vi "Import data part 1.vi"() -> (1 "New Qs":T1[](array[typedef]), 3 "canceled?":bool)   [LabVIEW 2013]
uses:
  TD - Data type.ctl
  qwtblvlib/TD Quantity.ctl
  qwtblvlib/QWTBLVLib.lvlib
panel:
  in  "note":string="This vi can import only from csv/dat files."
  out "data type":T2
  in  "next":bool
  in  "Cancel":bool
  in  "Data filename":path
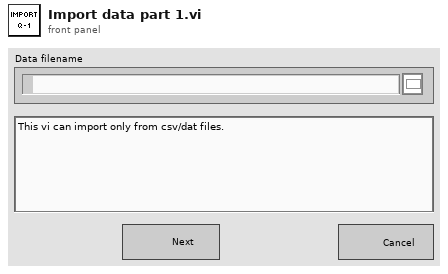
[diagram p1: front panel]
types:
  T1 = typedef "QWTBLVLib.lvlib/TD Quantity.ctl" = cluster{"Name":string, "Value":dbl[][], "Uncertainty":dbl[][], "Degrees of Freedom":dbl[][], "Correlation":dbl[][], "Randomized uncertainty":dbl[][]}
  T2 = typedef "TD - Data type.ctl" = enum32{"unknown", "csv", "xls/xlsx"}
  T3 = enum8{"Enabled", "Disabled", "Disabled and Grayed Out"}
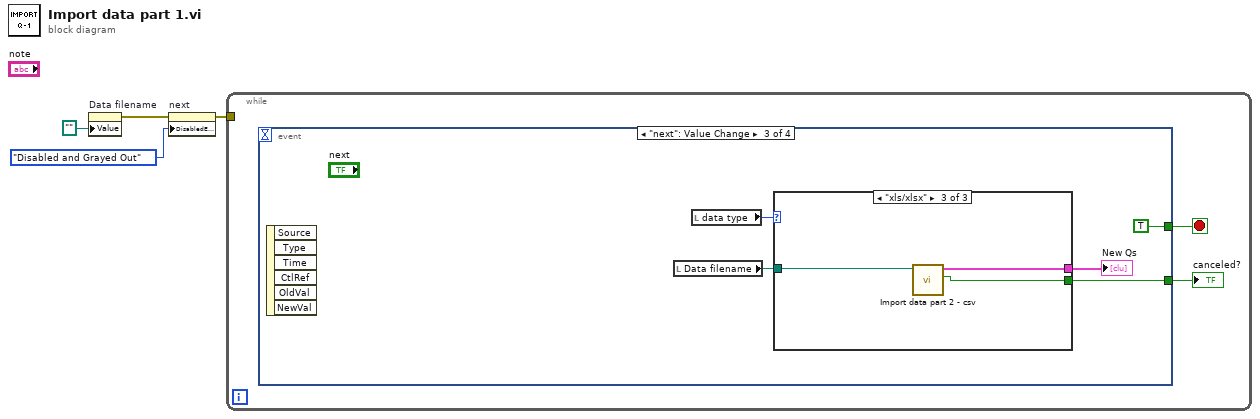
[diagram p0: block diagram]
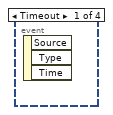
[diagram p2: hidden frame]
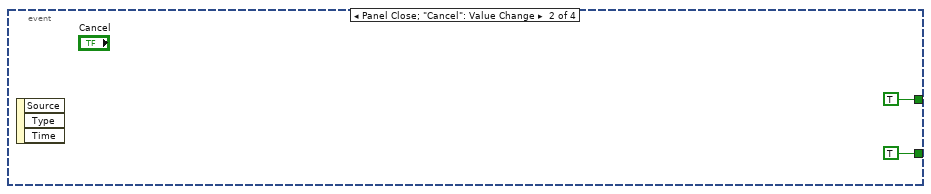
[diagram p3: hidden frame]
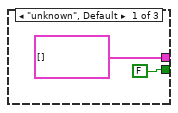
[diagram p4: hidden frame]
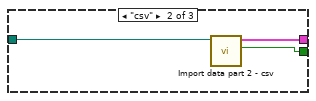
[diagram p5: hidden frame]
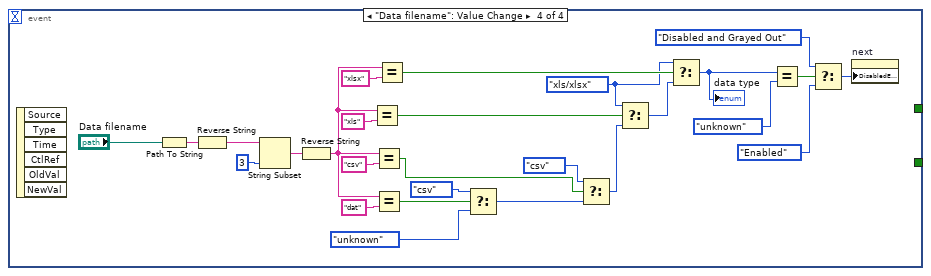
[diagram p6: hidden frame]
diagram:
  n1 = property on="Data filename" class="Path"("Value"=path "") -> (error out=w1:errorcluster)  [unwired: 2 in, 1 out]
  n2 = property on="next" class="Bool"(error in=w1, "DisabledEnum"=T3."Disabled and Grayed Out" ("Disabled")) -> (error out=w3:errorcluster)  [unwired: 1 in, 1 out]
  n3 = while {
    tunnel: w3 -> [_]
    stop <- w6 stop-if-true
    n4 = event shown="[2] \"next\": Value Change" {
      selector: _ -> [_ _ _ _]
      dyn-events: _ -> [_ _ _ _]
      timeout: _ -> [_ _ _ _]
      tunnel: [_ TRUE TRUE _] -> w6
      tunnel: [_ TRUE ("canceled") w10 _] -> w5
      event Timeout {
        n5 = event-data() -> ()  [unwired: 1 in, 3 out]
      }
      event Panel Close; "Cancel": Value Change {
        n6 = event-data() -> ()  [unwired: 1 in, 3 out]
      }
      event "next": Value Change {
        n7 = event-data() -> ()  [unwired: 1 in, 6 out]
        n8 = local read "Data filename"() -> (w13:path)
        n9 = local read "data type"() -> (w11:T2)
        n10 = case shown="\"xls/xlsx\"" w11 {
          tunnel: w13 -> [_ w18 w21]
          tunnel: [T1[] [] ("New Qs") w17 w20] -> w9
          tunnel: [FALSE ("canceled?") w16 w19] -> w10
          frame "unknown", Default {
          }
          frame "csv" {
            n11 = call "Import data part 2 - csv.vi"("Data filename"=w18) -> ("canceled?"=w16:bool, "New Qs"=w17:T1[])  [unwired: 7 in]
          }
          frame "xls/xlsx" {
            n12 = call "Import data part 2 - csv.vi"("Data filename"=w21) -> ("canceled?"=w19:bool, "New Qs"=w20:T1[])  [unwired: 7 in]
          }
        }
        "New Qs" <- w9
      }
      event "Data filename": Value Change {
        w31 = TD_-_Data_type."xls/xlsx" ("data type")
        n13 = event-data() -> ()  [unwired: 1 in, 6 out]
        n14 = Path To String(path="Data filename") -> (string=w47:string)
        n15 = Reverse String(1:w47) -> (0:w46:string)
        n16 = String Subset(string=w46, length (rest)=3 ("length (rest)")) -> (substring=w44:string)  [unwired: 1 in]
        n17 = Reverse String(1:w44) -> (0:w29:string)
        n18 = Equal?(x=w29, y="xls") -> (x = y?=w38:bool)
        n19 = Equal?(x=w29, y="csv") -> (x = y?=w37:bool)
        n20 = Equal?(x=w29, y="dat") -> (x = y?=w28:bool)
        n21 = Equal?(x=w29, y="xlsx") -> (x = y?=w36:bool)
        n22 = Select(t=TD_-_Data_type."csv" ("data type"), s=w28, f=TD_-_Data_type."unknown" ("data type")) -> (s? t:f=w25:T2)
        n23 = Select(t=TD_-_Data_type."csv" ("data type"), s=w37, f=w25) -> (s? t:f=w40:T2)
        n24 = Select(t=w31, s=w38, f=w40) -> (s? t:f=w39:T2)
        n25 = Select(t=w31, s=w36, f=w39) -> (s? t:f=w24:T2)
        "data type" <- w24
        n26 = Equal?(x=w24, y=TD_-_Data_type."unknown" ("data type")) -> (x = y?=w22:bool)
        n27 = Select(t=T3."Disabled and Grayed Out" ("Disabled"), s=w22, f=T3."Enabled" ("Disabled")) -> (s? t:f=w33:T3)
        n28 = property on="next" class="Bool"("DisabledEnum"=w33) -> ()  [unwired: 2 in, 2 out]
      }
    }
    "canceled?" <- w5
  }
